vi "ACQ enkoders to wfm.vi"(6 "Enk Chan Name":string[](array[string])=["Kana³ A", "Kana³ B"], 7 "data":waveform(dbl)[](array[waveform]), 8 "error in (no error)":errorcluster, 10 "Data Y":dbl[](array[numeric]), 11 "Data X":dbl[](array[numeric])) -> (0 "error out":errorcluster, 2 "Enk wfm out":waveform(dbl)[](array[waveform]))   [LabVIEW 2014]
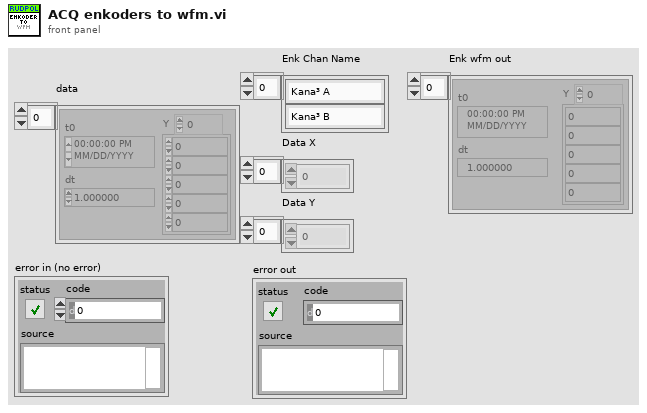
[diagram p1: front panel]
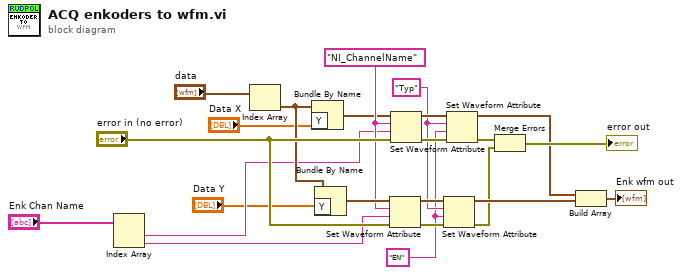
[diagram p0: block diagram]
diagram:
  w1 = "EN"
  w2 = "Typ"
  w21 = "NI_ChannelName" ("name")
  n1 = Index Array(array="Enk Chan Name") -> (element #1=w7:string, element #2=w6:string)  [unwired: 2 in]
  n2 = Index Array(array="data") -> (element=w20:waveform(dbl))  [unwired: 1 in]
  n3 = Bundle By Name(cluster=w20, "Y"="Data X") -> (w18:waveform(dbl))
  n4 = Bundle By Name(cluster=w20, "Y"="Data Y") -> (w22:waveform(dbl))
  n5 = Set Waveform Attribute(4:"error in (no error)", 5:w6, 6:w21, 7:w22) -> (0:w12:errorcluster, 3:w11:waveform(dbl))  [unwired: 1 out]
  n6 = Set Waveform Attribute(4:"error in (no error)", 5:w7, 6:w21, 7:w18) -> (0:w16:errorcluster, 3:w15:waveform(dbl))  [unwired: 1 out]
  n7 = Set Waveform Attribute(4:w12, 5:w1, 6:w2, 7:w11) -> (0:w9:errorcluster, 3:w10:waveform(dbl))  [unwired: 1 out]
  n8 = Set Waveform Attribute(4:w16, 5:w1, 6:w2, 7:w15) -> (0:w14:errorcluster, 3:w13:waveform(dbl))  [unwired: 1 out]
  n9 = Merge Errors(w14, w9) -> (→"error out":errorcluster)
  n10 = Build Array(w13, w10) -> (→"Enk wfm out":waveform(dbl)[])
